vi "Launcher.vi"() -> ()   [LabVIEW 2020]
uses:
  Controls/Currency Enum.ctl
  UI Actor/UI Actor.lvclass
  C:/Program Files (x86)/National Instruments/LabVIEW 2020/vi.lib/ActorFramework/Actor/Actor.lvclass
  UI Actor/UI Actor.lvclass/UI Actor.ctl
  UI Actor/Write Currency.vi
  <vilib>/ActorFramework/Actor/Actor.lvclass
panel:
  in  "Currency":T1 items=["USD", "MXN", "EUR"]
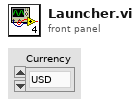
[diagram p1: front panel]
types:
  T1 = typedef "Currency Enum.ctl" = u16
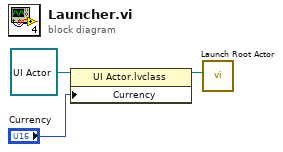
[diagram p0: block diagram]
diagram:
  n1 = property class="UI Actor.lvclass"(reference=refnum<class "UI Actor.lvclass"> refnum ("UI Actor.lvlib:UI Actor.lvclass"), "Currency"="Currency") -> (reference out=w2:refnum<class "UI Actor.lvclass">)  [unwired: 1 in, 1 out]
  n2 = call <vilib>:"Launch Root Actor.vi"("Actor"=w2) -> ()  [unwired: 9 in, 2 out]
